vi "Version Constant.vi"() -> ()   [LabVIEW 2014, in "base TBM sequencer configuration.lvclass"]
uses:
  base TBM sequencer configuration.lvclass
panel:
  in  "Version":string="1.0.0.0"
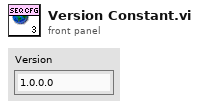
[diagram p1: front panel]
diagram:
